vi "ShowTheSpecifiedControl.vi"(7 "Command":T2(ring), 8 "index":i32, 11 "Ref Cluster":T1) -> (3 "element":refnum<vi>)   [LabVIEW 2017]
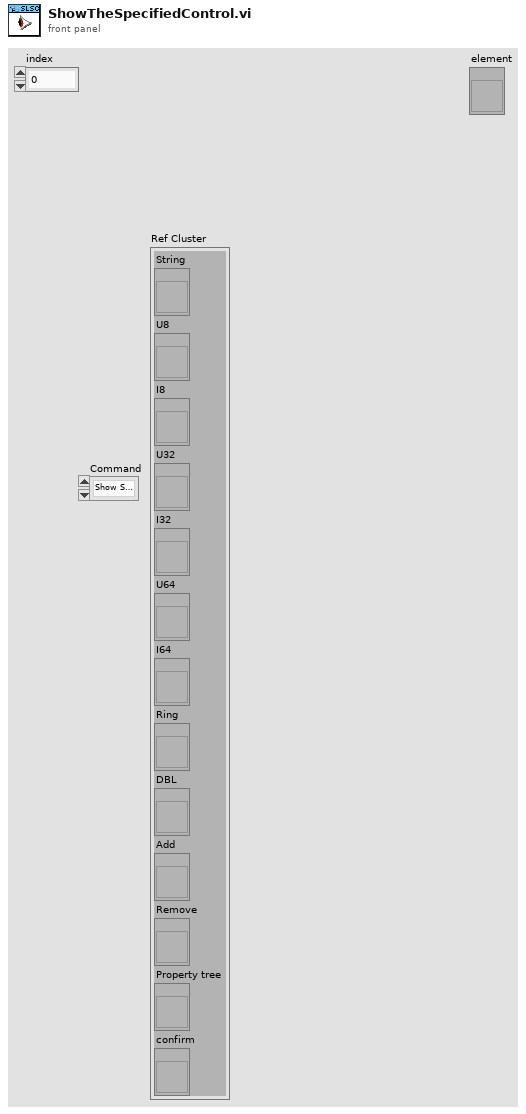
[diagram p1: front panel]
types:
  T1 = cluster{"String":refnum<vi>, "U8":refnum<vi>, "I8":refnum<vi>, "U32":refnum<vi>, "I32":refnum<vi>, "U64":refnum<vi>, "I64":refnum<vi>, "Ring":refnum<vi>, "DBL":refnum<vi>, "Add":refnum<vi>, "Remove":refnum<vi>, "Property tree":refnum<vi>, "confirm":refnum<vi>}
  T2 = enum16{"Show Selected Control", "All Visiable", "All Invisible"}
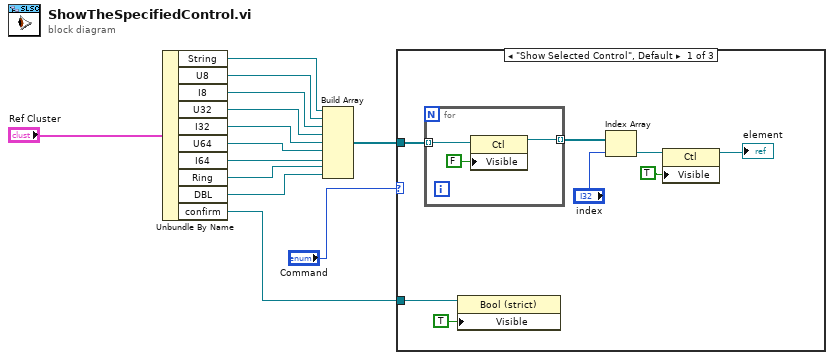
[diagram p0: block diagram]
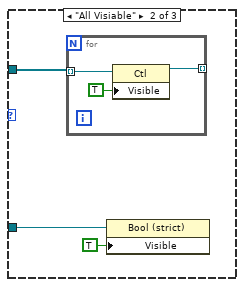
[diagram p2: hidden frame]
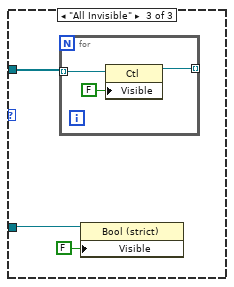
[diagram p3: hidden frame]
diagram:
  n1 = Unbundle By Name("Ref Cluster") -> ("String"=w5:refnum<vi>, "U8"=w6:refnum<vi>, "I8"=w7:refnum<vi>, "U32"=w8:refnum<vi>, "I32"=w9:refnum<vi>, "U64"=w10:refnum<vi>, "I64"=w11:refnum<vi>, "Ring"=w12:refnum<vi>, "DBL"=w4:refnum<vi>, "confirm"=w1:refnum<vi>)
  n2 = Build Array(w5, w6, w7, w8, w9, w10, w11, w12, w4) -> (w13:refnum<vi>[])
  n3 = case shown="\"Show Selected Control\", Default" "Command" {
    tunnel: w13 -> [w20 w26 w32]
    tunnel: w1 -> [w15 w25 w31]
    frame "Show Selected Control", Default {
      n4 = for {
        tunnel: w20 -> [w23] mode=indexing
        tunnel: [w21] -> w19 mode=indexing
        n5 = property class="Ctl"(reference=w23, "Visible"=FALSE) -> (reference out=w21:refnum<vi>)  [unwired: 1 in, 1 out]
      }
      n6 = property class="Bool (strict)"(reference=w15, "Visible"=TRUE) -> ()  [unwired: 1 in, 2 out]
      n7 = Index Array(array=w19, index="index") -> (element=w17:refnum<vi>)
      "element" <- w17
      n8 = property class="Ctl"(reference=w17, "Visible"=TRUE) -> ()  [unwired: 1 in, 2 out]
    }
    frame "All Visiable" {
      n9 = for {
        tunnel: w26 -> [w29] mode=indexing
        tunnel: [w27] -> _ mode=indexing
        n10 = property class="Ctl"(reference=w29, "Visible"=TRUE) -> (reference out=w27:refnum<vi>)  [unwired: 1 in, 1 out]
      }
      n11 = property class="Bool (strict)"(reference=w25, "Visible"=TRUE) -> ()  [unwired: 1 in, 2 out]
    }
    frame "All Invisible" {
      n12 = for {
        tunnel: w32 -> [w35] mode=indexing
        tunnel: [w33] -> _ mode=indexing
        n13 = property class="Ctl"(reference=w35, "Visible"=FALSE) -> (reference out=w33:refnum<vi>)  [unwired: 1 in, 1 out]
      }
      n14 = property class="Bool (strict)"(reference=w31, "Visible"=FALSE) -> ()  [unwired: 1 in, 2 out]
    }
  }
